vi "Read Server Generic UE.vi"(11 "Template Server in":refnum<class "Template Server.lvclass">) -> (2 "Server Generic UE":refnum<user-event>, 3 "Template Server out":refnum<class "Template Server.lvclass">)   [LabVIEW 2019, in "Template Server.lvlib" / "Template Server.lvclass"]
uses:
  Template Server.lvclass
  <vilib>/gRPC/LabVIEW gRPC Library/Server API/typeDefs/Generic Method Event Data.ctl
  <vilib>/gRPC/LabVIEW gRPC Library/Shared/grpcId.ctl
  Template Server.lvclass/Template Server.ctl
  <vilib>/gRPC/LabVIEW gRPC Library/grpc-lvsupport-release.lvlib
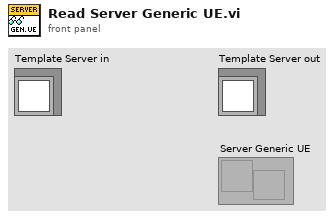
[diagram p1: front panel]
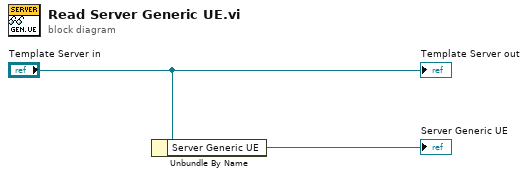
[diagram p0: block diagram]
diagram:
  n1 = Unbundle By Name("Template Server in") -> ("Server Generic UE"=→"Server Generic UE":refnum<user-event>)
  "Template Server out" <- "Template Server in"
